vi "ListDevicesSandbox.vi"() -> ()   [LabVIEW 2019]
uses:
  src/DAQmx/typedefs/DeviceInfo--Cluster.ctl
  <vilib>/nisyscfg/Filter Mode.ctl
  <vilib>/nisyscfg/Close (Filter).vi
  <vilib>/nisyscfg/Close (Hardware).vi
  <vilib>/nisyscfg/Close (System).vi
  src/DAQmx/DAQmx.lvclass
  <resource>/objmgr/nicontrollersysapi.rc
  <vilib>/nisyscfg/nisyscfg.lvlib
  <resource>/objmgr/nisysapi.rc
  <resource>/objmgr/daqmx.rc
panel:
  out "cal due?":bool
  in  "error in (no error) 2":errorcluster
  out "error out 2":errorcluster
  out "Devices":T1[](array[typedef])
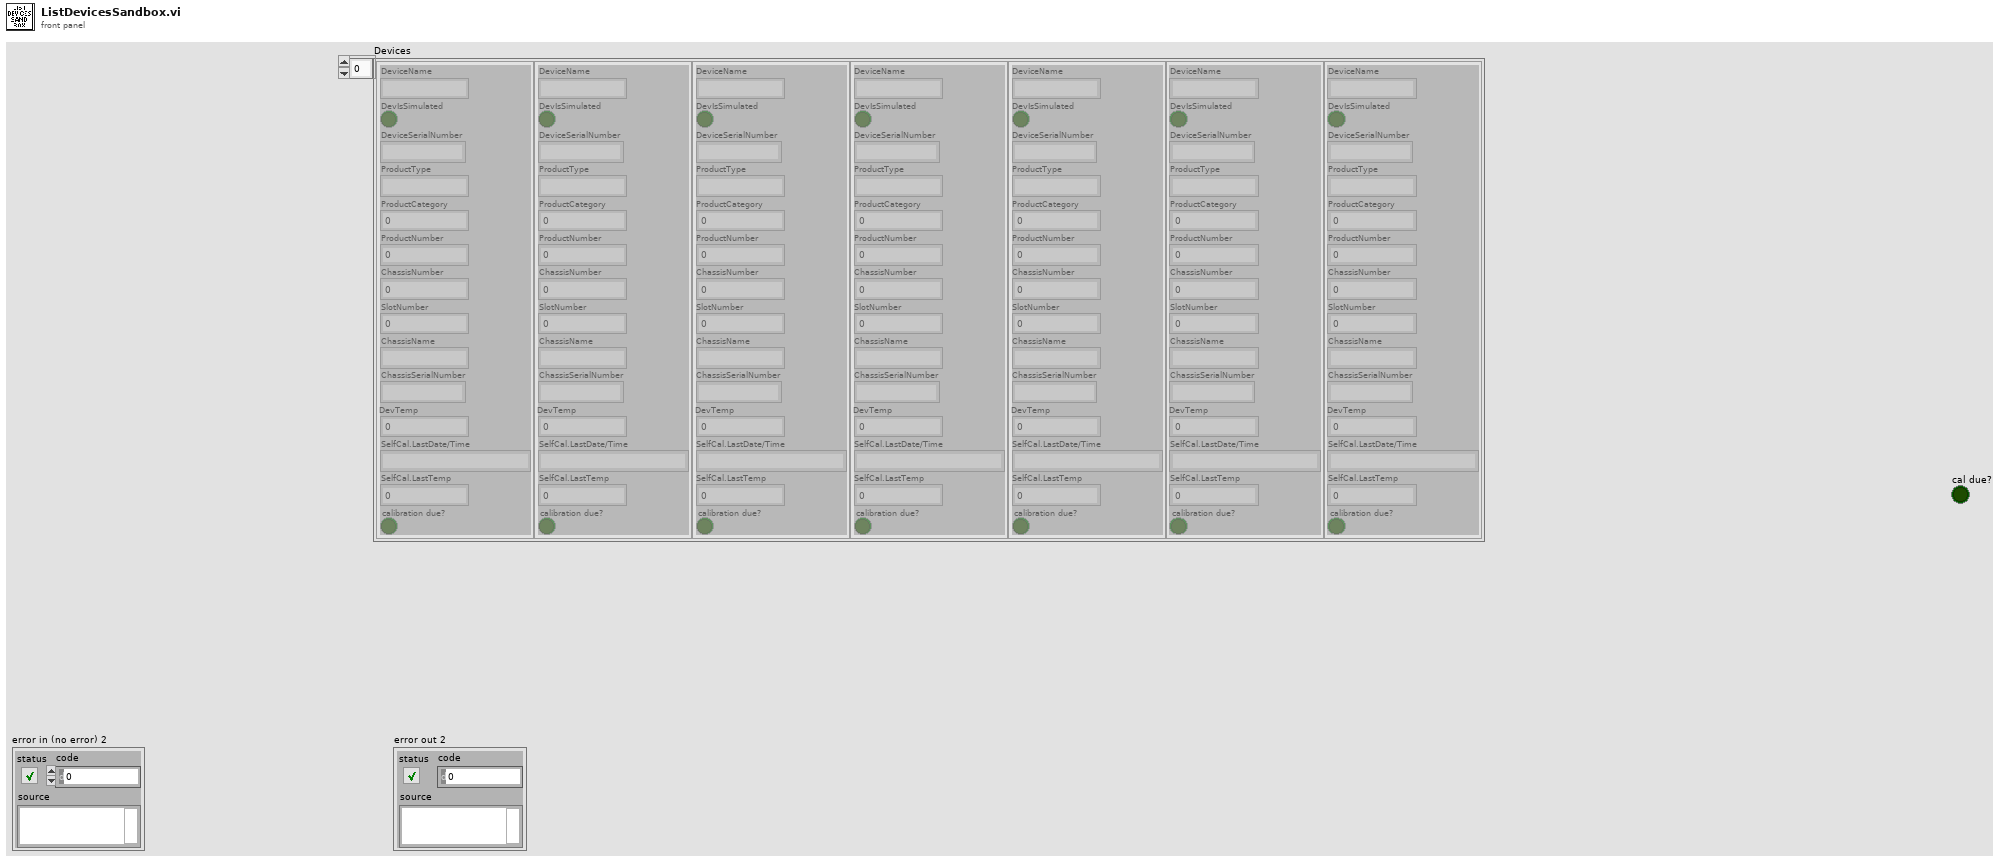
[diagram p1: front panel]
types:
  T1 = typedef "DAQmx.lvclass/DeviceInfo--Cluster.ctl" = cluster{"DeviceName":string, "DevIsSimulated":bool, "DeviceSerialNumber":string, "ProductType":string, "ProductCategory":i32, "ProductNumber":u32, "ChassisNumber":u32, "SlotNumber":u32, "ChassisName":string, "ChassisSerialNumber":string, "DevTemp":dbl, "SelfCal.LastDate/Time":string, "SelfCal.LastTemp":dbl, "calibration due?":bool}
  T2 = typedef "nisyscfg.lvlib/Filter Mode.ctl" = i32
  T3 = cluster{"Active Device":string, "SelfCal.LastDate/Time":string, "SelfCal.LastTemp":dbl, "DevTemp":dbl, "calibration due?":bool}
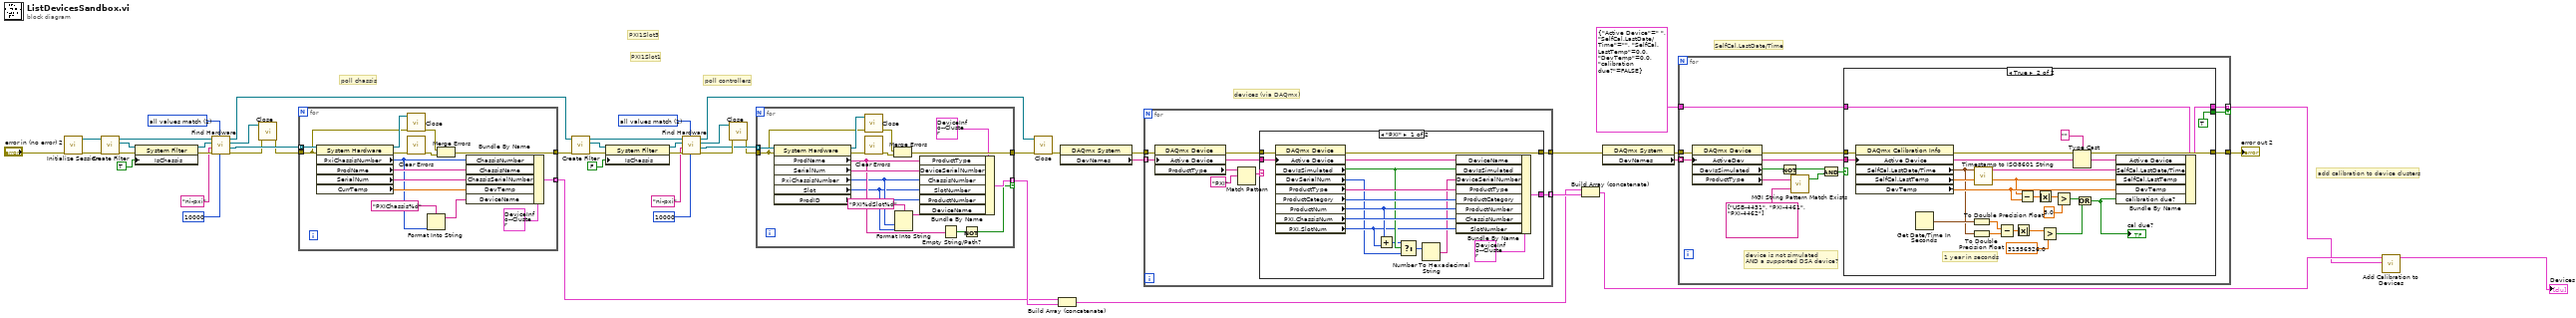
[diagram p0: block diagram]
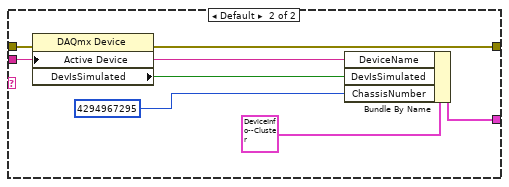
[diagram p2: hidden frame]
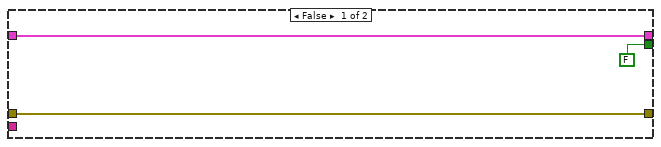
[diagram p3: hidden frame]
diagram:
  w24 = T2 1 items=["all values match"=1, "any value matches"=2, "values do not match"=3, "all properties exist"=4] ("Filter Mode (all values match)")
  w33 = T2 1 items=["all values match"=1, "any value matches"=2, "values do not match"=3, "all properties exist"=4] ("Filter Mode (all values match)")
  # "add calibration to device clusters"
  # "devices (via DAQmx)"
  # "poll controllers"
  # "poll chassis"
  # "PXI1Slot1"
  # "PXI1Slot3"
  # "SelfCal.LastDate/Time"
  n1 = call <vilib>:"Initialize Session.vi"("error in (no error)"="error in (no error) 2") -> ("error out"=w31:errorcluster, "Session out"=w32:refnum<k21>)  [unwired: 9 in]
  n2 = call <vilib>:"Create Filter.vi"("error in (no error)"=w31, "Session in"=w32) -> ("error out"=w40:errorcluster, "Filter out"=w39:refnum<k20>, "Session out"=w38:refnum<k21>)  [unwired: 7 in]
  n3 = property class="System Filter"(reference=w39, error in=w40, "IsChassis"=TRUE ("Is Chassis")) -> (reference out=w37:refnum<k20>, error out=w36:errorcluster)
  n4 = call <vilib>:"Find Hardware.vi"("Remote Timeout (300,000 ms)"=u32 10000, "Filter Mode (all values match)"=w33, "error in (no error)"=w36, "Experts"="ni-pxi", "Filter in"=w37, "Session in"=w38) -> ("error out"=w29:errorcluster, "Resources out"=w41:refnum<k20>[], "Filter out"=w30:refnum<k20>, "Session out"=w15:refnum<k21>)  [unwired: 2 in]
  n5 = call-poly <vilib>:"Close.vi"("error in (no error)"=w29, "Filter in"=w30) -> ("error out"=w28:errorcluster)  [unwired: 9 in]
  n6 = for {
    tunnel: w41 -> [w63] mode=indexing
    tunnel: w28 -> [w58]
    tunnel: [w61] -> w16
    tunnel: [w54] -> w3 mode=indexing
    n7 = property class="System Hardware"(reference=w63, error in=w58) -> (reference out=w62:refnum<k20>, error out=w60:errorcluster, "PxiChassisNumber"=w51:u32, "ProdName"=w56:string, "SerialNum"=w53:string, "CurrTemp"=w52:dbl)
    n8 = call-poly <vilib>:"Close.vi"("error in (no error)"=w58, "Resource in"=w62) -> ("error out"=w59:errorcluster)  [unwired: 9 in]
    n9 = call <vilib>:"Clear Errors.vi"("error in (no error)"=w60) -> ("error out"=w57:errorcluster)  [unwired: 5 in, 1 out]
    n10 = Format Into String(format string="PXIChassis%d" ("DeviceName"), w51) -> (resulting string=w49:string)  [unwired: 2 in, 1 out]
    n11 = Merge Errors(w59, w57) -> (w61:errorcluster)
    n12 = Bundle By Name(cluster=T1 {"DeviceName"="", "DevIsSimulated"=FALSE, "DeviceSerialNumber"="", "ProductType"="", "ProductCategory"=0, "ProductNumber"=0, "ChassisNumber"=0, "SlotNumber"=0, "ChassisName"="", "ChassisSerialNumber"="", "DevTemp"=0.0, "SelfCal.LastDate/Time"="", "SelfCal.LastTemp"=0.0, "calibration due?"=FALSE} ("Device"), "ChassisNumber"=w51, "ChassisName"=w56, "ChassisSerialNumber"=w53, "DevTemp"=w52, "DeviceName"=w49) -> (w54:T1)
  }
  n13 = call <vilib>:"Create Filter.vi"("error in (no error)"=w16, "Session in"=w15) -> ("error out"=w18:errorcluster, "Filter out"=w19:refnum<k20>, "Session out"=w20:refnum<k21>)  [unwired: 7 in]
  n14 = property class="System Filter"(reference=w19, error in=w18, "IsChassis"=FALSE ("Is Chassis")) -> (reference out=w21:refnum<k20>, error out=w22:errorcluster)
  n15 = call <vilib>:"Find Hardware.vi"("Remote Timeout (300,000 ms)"=u32 10000, "Filter Mode (all values match)"=w24, "error in (no error)"=w22, "Experts"="ni-pxi", "Filter in"=w21, "Session in"=w20) -> ("error out"=w26:errorcluster, "Resources out"=w13:refnum<k20>[], "Filter out"=w25:refnum<k20>, "Session out"=w14:refnum<k21>)  [unwired: 2 in]
  n16 = call-poly <vilib>:"Close.vi"("error in (no error)"=w26, "Filter in"=w25) -> ("error out"=w12:errorcluster)  [unwired: 9 in]
  n17 = for {
    tunnel: w13 -> [w81] mode=indexing
    tunnel: w12 -> [w76]
    tunnel: [w79] -> w11
    tunnel: [w72] -> w5 mode=indexing if=w69
    n18 = property class="System Hardware"(reference=w81, error in=w76) -> (reference out=w80:refnum<k20>, error out=w78:errorcluster, "ProdName"=w71:string, "SerialNum"=w73:string, "PxiChassisNumber"=w66:u32, "Slot"=w65:i32, "ProdID"=w68:u32)
    n19 = call-poly <vilib>:"Close.vi"("error in (no error)"=w76, "Resource in"=w80) -> ("error out"=w77:errorcluster)  [unwired: 9 in]
    n20 = call <vilib>:"Clear Errors.vi"("error in (no error)"=w78) -> ("error out"=w75:errorcluster)  [unwired: 5 in, 1 out]
    n21 = Merge Errors(w77, w75) -> (w79:errorcluster)
    n22 = Format Into String(format string="PXI%dSlot%d" ("DeviceName"), w66, w65) -> (resulting string=w64:string)  [unwired: 2 in, 1 out]
    n23 = Bundle By Name(cluster=T1 {"DeviceName"="", "DevIsSimulated"=FALSE, "DeviceSerialNumber"="", "ProductType"="", "ProductCategory"=0, "ProductNumber"=0, "ChassisNumber"=0, "SlotNumber"=0, "ChassisName"="", "ChassisSerialNumber"="", "DevTemp"=0.0, "SelfCal.LastDate/Time"="", "SelfCal.LastTemp"=0.0, "calibration due?"=FALSE} ("Device"), "ProductType"=w71, "DeviceSerialNumber"=w73, "ChassisNumber"=w66, "SlotNumber"=w65, "ProductNumber"=w68, "DeviceName"=w64) -> (w72:T1)
    n24 = Empty String/Path?(string/path=w71) -> (empty?=w70:bool)
    n25 = Not(x=w70) -> (.not. x?=w69:bool)
  }
  n26 = call-poly <vilib>:"Close.vi"("error in (no error)"=w11, "Session in"=w14) -> ("error out"=w7:errorcluster)  [unwired: 9 in]
  n27 = Build Array (concatenate)(w3, w5) -> (w4:T1[])
  n28 = property class="DAQmx System"(error in=w7) -> (error out=w9:errorcluster, "DevNames"=w10:tag[])  [unwired: 1 in, 1 out]
  n29 = for {
    tunnel: w10 -> [w83] mode=indexing
    tunnel: w9 -> [w89]
    tunnel: [w84] -> w45
    tunnel: [w82] -> w8 mode=indexing
    n30 = property class="DAQmx Device"(error in=w89, "Active Device"=w83) -> (error out=w85:errorcluster, "ProductType"=w88:string)  [unwired: 1 in, 1 out]
    n31 = Match Pattern(string=w88, regular expression="PXI") -> (match substring=w87:string)  [unwired: 1 in, 3 out]
    n32 = case shown="\"PXI\"" w87 {
      tunnel: w85 -> [w104 w110]
      tunnel: [w103 w111] -> w84
      tunnel: w83 -> [w102 w108]
      tunnel: [w101 w105] -> w82
      frame "PXI" {
        n33 = property class="DAQmx Device"(error in=w104, "Active Device"=w102) -> (error out=w103:errorcluster, "DevIsSimulated"=w95:bool, "DevSerialNum"=w92:u32, "ProductType"=w97:string, "ProductCategory"=w98:i32, "ProductNum"=w96:u32, "PXI.ChassisNum"=w99:u32, "PXI.SlotNum"=w93:u32)  [unwired: 1 in, 1 out]
        n34 = Add(x=w96, y=w93) -> (x+y=w94:u32)
        n35 = Select(t=w94, s=w95, f=w92) -> (s? t:f=w91:u32)
        n36 = Number To Hexadecimal String(2:w91) -> (0:w90:string)  [unwired: 1 in]
        n37 = Bundle By Name(cluster=T1 {"DeviceName"="", "DevIsSimulated"=FALSE, "DeviceSerialNumber"="", "ProductType"="", "ProductCategory"=0, "ProductNumber"=0, "ChassisNumber"=0, "SlotNumber"=0, "ChassisName"="", "ChassisSerialNumber"="", "DevTemp"=0.0, "SelfCal.LastDate/Time"="", "SelfCal.LastTemp"=0.0, "calibration due?"=FALSE} ("Device"), "DeviceName"=w102, "DevIsSimulated"=w95, "DeviceSerialNumber"=w90, "ProductType"=w97, "ProductCategory"=w98, "ProductNumber"=w96, "ChassisNumber"=w99, "SlotNumber"=w93) -> (w101:T1)
      }
      frame Default {
        n38 = property class="DAQmx Device"(error in=w110, "Active Device"=w108) -> (error out=w111:errorcluster, "DevIsSimulated"=w107:bool)  [unwired: 1 in, 1 out]
        n39 = Bundle By Name(cluster=T1 {"DeviceName"="", "DevIsSimulated"=FALSE, "DeviceSerialNumber"="", "ProductType"="", "ProductCategory"=0, "ProductNumber"=0, "ChassisNumber"=0, "SlotNumber"=0, "ChassisName"="", "ChassisSerialNumber"="", "DevTemp"=0.0, "SelfCal.LastDate/Time"="", "SelfCal.LastTemp"=0.0, "calibration due?"=FALSE} ("Device"), "DeviceName"=w108, "DevIsSimulated"=w107, "ChassisNumber"=u32 4294967295 ("PXI.ChassisNum")) -> (w105:T1)
      }
    }
  }
  n40 = Build Array (concatenate)(w4, w8) -> (w2:T1[])
  n41 = property class="DAQmx System"(error in=w45) -> (error out=w47:errorcluster, "DevNames"=w48:tag[])  [unwired: 1 in, 1 out]
  n42 = for {
    tunnel: [w123] -> w1 mode=indexing if=w114
    tunnel: w48 -> [w121] mode=indexing
    tunnel: T3 {"Active Device"=" ", "SelfCal.LastDate/Time"="", "SelfCal.LastTemp"=0.0, "DevTemp"=0.0, "calibration due?"=FALSE} ("element") -> [w112]
    tunnel: w47 -> [w122]
    tunnel: [w124] -> w44
    # "device is not simulated\nAND a supported DSA device?"
    n43 = property class="DAQmx Device"(error in=w122, "ActiveDev"=w121) -> (error out=w120:errorcluster, "DevIsSimulated"=w119:bool, "ProductType"=w116:string)  [unwired: 1 in, 1 out]
    n44 = Not(x=w119) -> (.not. x?=w117:bool)
    n45 = call <userlib>:"MGI String Pattern Match Exists.vi"("Patterns to Try"=string[] ["USB-4431", "PXI-4461", "PXI-4462"], "String"=w116) -> ("Match Found"=w115:bool)  [unwired: 1 out]
    n46 = And(x=w117, y=w115) -> (x .and. y?=w118:bool)
    n47 = case shown="True" w118 {
      tunnel: [w127 w151] -> w124
      tunnel: [w125 w138] -> w123
      tunnel: w121 -> [_ w140]
      tunnel: w120 -> [w127 w139]
      tunnel: [FALSE TRUE] -> w114
      tunnel: w112 -> [w125 w137]
      frame False {
      }
      frame True {
        # "1 year in seconds"
        n48 = property class="DAQmx Calibration Info"(error in=w139, "Active Device"=w140) -> (error out=w151:errorcluster, "SelfCal.LastDate/Time"=w128:timestamp, "SelfCal.LastTemp"=w146:dbl, "DevTemp"=w147:dbl)  [unwired: 1 in, 1 out]
        n49 = Get Date/Time In Seconds() -> (seconds since 1Jan1904=w134:timestamp)
        n50 = To Double Precision Float(number=w134) -> (double precision float=w132:dbl)
        n51 = To Double Precision Float(number=w128) -> (double precision float=w133:dbl)
        n52 = call <vilib>:"Timestamp to ISO8601 String.vi"("Timestamp (now)"=w128) -> ("ISO8601 String"=w129:string)  [unwired: 10 in]
        n53 = Subtract(x=w132, y=w133) -> (x-y=w145:dbl)
        n54 = Absolute Value(x=w145) -> (abs(x)=w144:dbl)
        n55 = Subtract(x=w146, y=w147) -> (x-y=w150:dbl)
        n56 = Absolute Value(x=w150) -> (abs(x)=w149:dbl)
        n57 = Greater?(x=w144, y=31556926.0) -> (0:w142:bool)
        n58 = Greater?(x=w149, y=5.0) -> (0:w143:bool)
        n59 = Type Cast(type="", x=w140) -> (*(type *) &x=w131:string)
        n60 = Or(x=w143, y=w142) -> (x .or. y?=w135:bool)
        "cal due?" <- w135
        n61 = Bundle By Name(cluster=w137, "Active Device"=w131, "SelfCal.LastDate/Time"=w129, "SelfCal.LastTemp"=w146, "DevTemp"=w147, "calibration due?"=w135) -> (w138:T3)
      }
    }
  }
  "error out 2" <- w44
  n62 = call "Add Calibration to Devices.vi"("Calibration in"=w1, "Devices in"=w2) -> ("Devices out"=→"Devices":T1[])  [unwired: 9 in]
